vi "Calibration profile data column headers.vi"(8 "error in (no error)":errorcluster) -> (0 "error out":errorcluster, 1 "File headers":string[](array[string]), 2 "Col Hdrs Full":string[](array[string]), 3 "Col Hdrs Trunc.":string[](array[string]))   [LabVIEW 2020]
uses:
  TypeDefs/Current Imaging Parameters.ctl
  TypeDefs/Current Calibration Parameters.ctl
panel:
  out "Units array":string[](array[string])
  in  "Units":string[](array[string])=["val", "val", "val", "val", "val", "gain", "gain", "cycles", "cycles", "nm"]
  in  "Units":string[](array[string])=["µm", "µm", "µm", "µm", "µm", "µm", "µm", "µS", "pixels", "gain", "deg", "deg", "deg", "%", "gain val", "gain val"]
  in  "Current Calibration Parameters":T1={"Sum X"=0.0, "Sum Y"=0.0, "Diff X"=0.0, "Diff Y"=0.0, "Distortion Correction"=0.0, "Z_norm to um_scaling"=0.0, "X_norm to um_scaling"=0.0, "Samples to Wait after Trigger"=0.0, "Slip Cycle"=0.0, "Calibration Wavelength"=2.0}
  out "Array 2":string[](array[string])
  out "Hdrs":string[](array[string])
  in  "Calibration-Imaging Parameters":T2
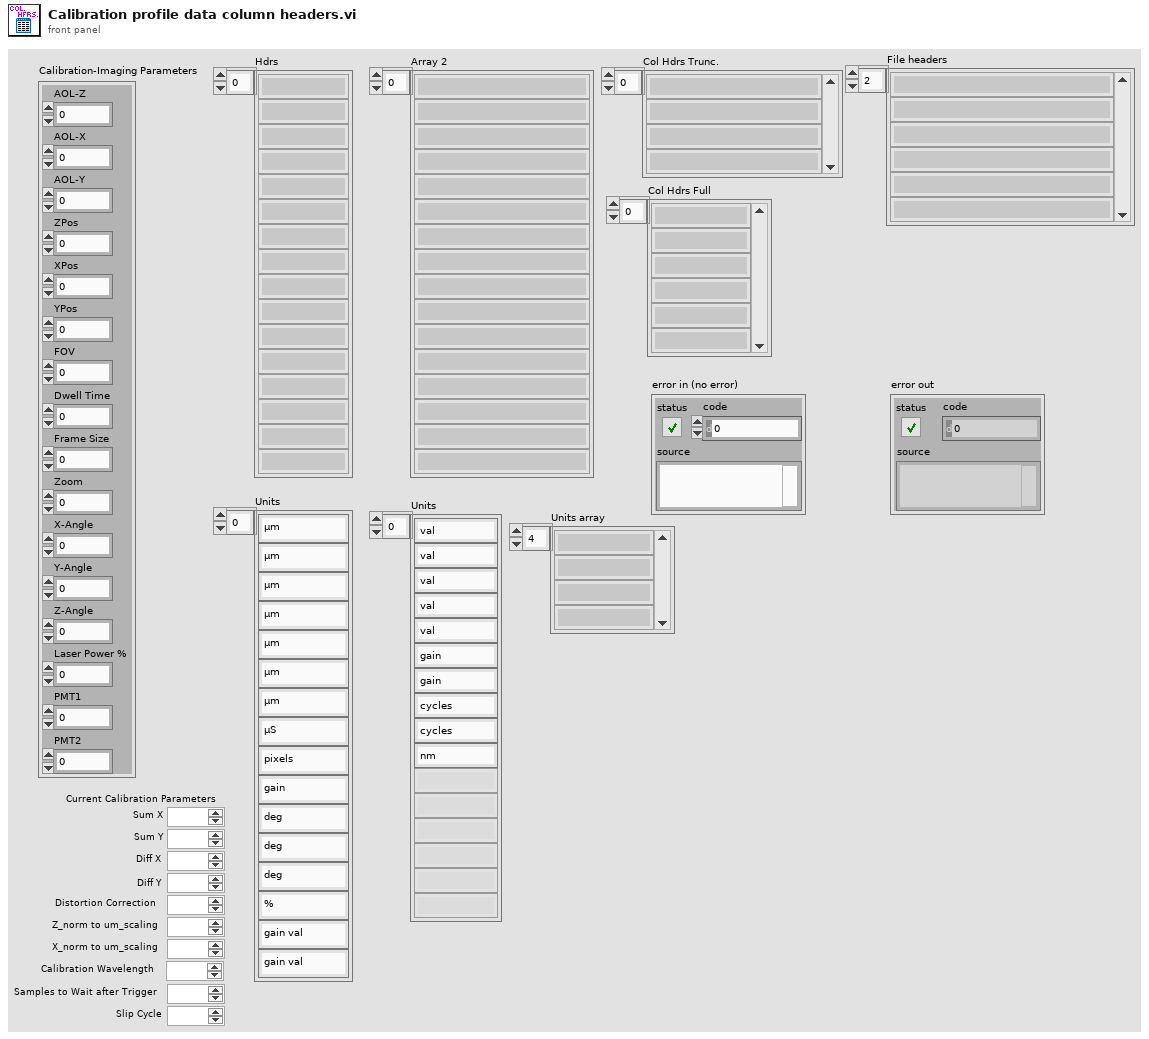
[diagram p1: front panel]
types:
  T1 = typedef "Current Calibration Parameters.ctl" = cluster{"Sum X":dbl, "Sum Y":dbl, "Diff X":dbl, "Diff Y":dbl, "Distortion Correction":dbl, "Z_norm to um_scaling":dbl, "X_norm to um_scaling":dbl, "Samples to Wait after Trigger":dbl, "Slip Cycle":dbl, "Calibration Wavelength":dbl}
  T2 = typedef "Current Imaging Parameters.ctl" = cluster{"AOL-Z":dbl, "AOL-X":dbl, "AOL-Y":dbl, "ZPos":dbl, "XPos":dbl, "YPos":dbl, "FOV":dbl, "Dwell Time":dbl, "Frame Size":dbl, "Zoom":dbl, "X-Angle":dbl, "Y-Angle":dbl, "Z-Angle":dbl, "Laser Power %":dbl, "PMT1":dbl, "PMT2":dbl}
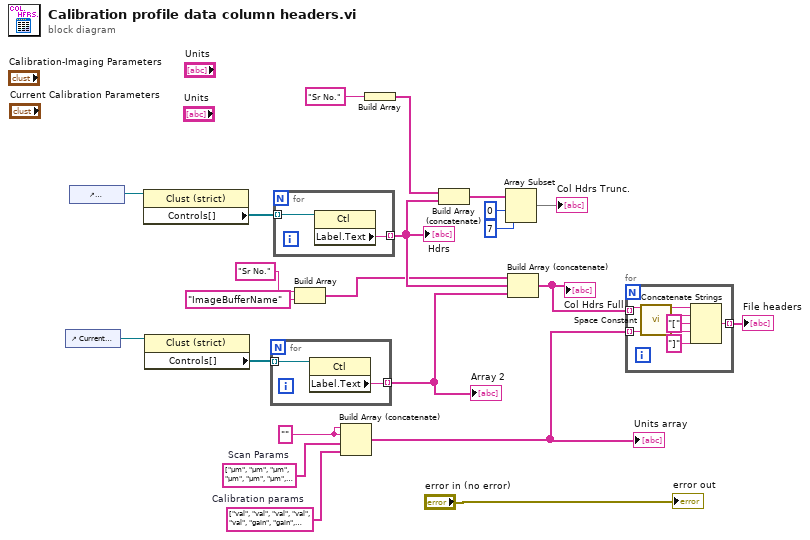
[diagram p0: block diagram]
diagram:
  w1 = ""
  w12 = string[] ["val", "val", "val", "val", "val", "gain", "gain", "cycles", "cycles", "nm"]  # Calibration params
  w13 = string[] ["µm", "µm", "µm", "µm", "µm", "µm", "µm", "µS", "pixels", "gain", "deg", "deg", "deg", "%", "gain val", "gain val"]  # Scan Params
  n1 = control-ref of="Current Calibration Parameters"() -> (w19:refnum<vi>)
  n2 = control-ref of="Calibration-Imaging Parameters"() -> (w22:refnum<vi>)
  n3 = property class="Clust (strict)"(reference=w22) -> ("Controls[]"=w21:refnum<vi>[])  [unwired: 1 in, 2 out]
  n4 = property class="Clust (strict)"(reference=w19) -> ("Controls[]"=w20:refnum<vi>[])  [unwired: 1 in, 2 out]
  n5 = for {
    tunnel: w20 -> [w24] mode=indexing
    tunnel: [w23] -> w8 mode=indexing
    n6 = property class="Ctl"(reference=w24) -> ("Label.Text"=w23:string)  [unwired: 1 in, 2 out]
  }
  "Array 2" <- w8
  n7 = for {
    tunnel: w21 -> [w26] mode=indexing
    tunnel: [w25] -> w6 mode=indexing
    n8 = property class="Ctl"(reference=w26) -> ("Label.Text"=w25:string)  [unwired: 1 in, 2 out]
  }
  "Hdrs" <- w6
  n9 = Build Array("Sr No.", "ImageBufferName" ("element")) -> (w3:string[])
  n10 = Build Array (concatenate)(w1, w1, w13, w12) -> (w11:string[])
  "Units array" <- w11
  n11 = Build Array("Sr No.") -> (w17:string[])
  n12 = Build Array (concatenate)(w17, w6) -> (w9:string[])
  n13 = Array Subset(array=w9, index=0, length=7) -> (→"Col Hdrs Trunc.":string[])
  n14 = Build Array (concatenate)(w3, w6, w8) -> (w7:string[])
  "Col Hdrs Full" <- w7
  n15 = for {
    tunnel: w7 -> [w32] mode=indexing
    tunnel: w11 -> [w29] mode=indexing
    tunnel: [w27] -> w10 mode=indexing
    n16 = call <vilib>:"Space Constant.vi"() -> ("String"=w31:string)
    n17 = Concatenate Strings(w32, w31, "[" ("string"), w29, "]" ("string")) -> (w27:string)
  }
  "File headers" <- w10
  "error out" <- "error in (no error)"
